vi "From Scratch.vi"() -> ()   [LabVIEW 2020]
uses:
  <vilib>/userdefined/High Color/IMAQdx.ctl
  <vilib>/vision/driver/IMAQdx.llb/IMAQdx Acquisition Mode.ctl
  <vilib>/vision/driver/IMAQdx.llb/IMAQdx Buffer Number Mode.ctl
  <vilib>/vision/driver/NI_Vision_Acquisition_Software.lvlib
  <resource>/objmgr/imaqdx.rc
panel:
  in  "Stop Stream":bool
  in  "Simulated Processing Delay (ms)":i32
  out "Buffer Number Out":u32
  out "Images Missed":u32
  out "Images Behind":i32
  out "Processed Frames per Second":dbl
  out "Acquired Frames per Second":dbl
  out "Image":T1(plugin-control)
  in  "Number of Images (err Iteration)":i32
  in  "OverwriteMode":u16(ring) items=["Get Oldest"=0, "Fail"=2, "Get Newest"=3]
  in  "IMAQdx Session":T2
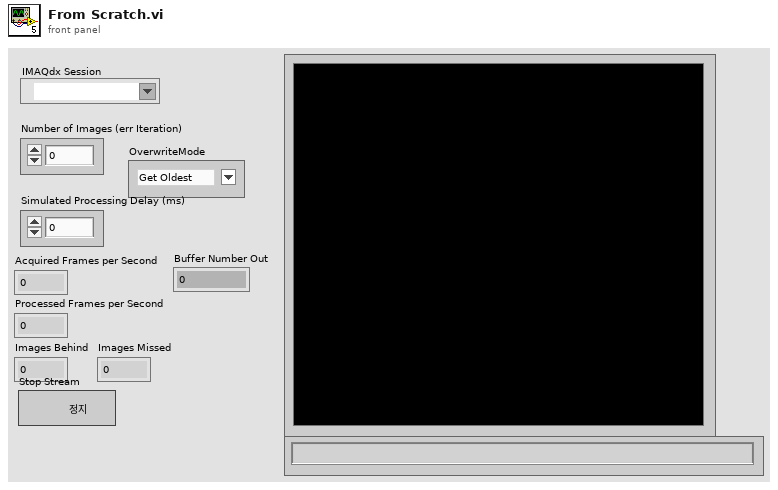
[diagram p1: front panel]
types:
  T1 = typedef "IMAQ Image.ctl" = refnum<image>
  T2 = typedef "IMAQdx.ctl" = refnum<k21>
  T3 = typedef "NI_Vision_Acquisition_Software.lvlib/IMAQdx Acquisition Mode.ctl" = enum32{"One Shot", "Continuous"}
  T4 = typedef "NI_Vision_Acquisition_Software.lvlib/IMAQdx Buffer Number Mode.ctl" = enum32{"Next", "Last", "Buffer Number", "Every", "Last New"}
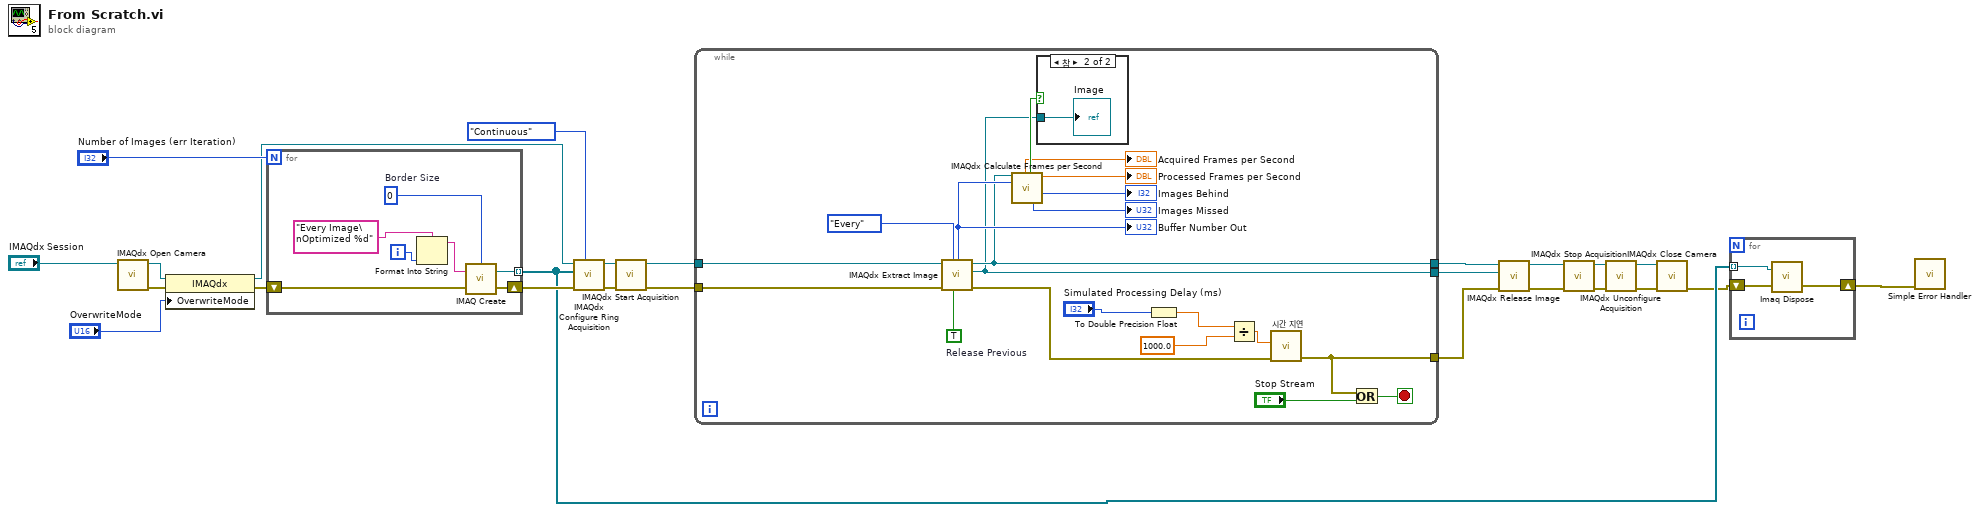
[diagram p0: block diagram]
diagram:
  n1 = call <vilib>:"IMAQdx Open Camera.vi"("Session In"="IMAQdx Session") -> ("error out"=w23:errorcluster, "Session Out"=w24:T2)  [unwired: 9 in]
  n2 = property class="IMAQdx"(reference=w24, error in=w23, "OverwriteMode"="OverwriteMode") -> (reference out=w18:T2, error out=w20:errorcluster)
  n3 = for {
    N: "Number of Images (err Iteration)" -> [_]
    tunnel: [w28] -> w3 mode=indexing
    shift-right: [w26] -> w17
    shift-left: w20 -> [w27]
    i -> [w31]
    w29 = 0  # Border Size
    n4 = Format Into String(format string="Every Image\nOptimized %d", w31) -> (resulting string=w30:string)  [unwired: 2 in, 1 out]
    n5 = call "IMAQ Create"("Border Size"=w29, "Image Name"=w30, "error in (no error)"=w27) -> ("New Image"=w28:T1, "error out"=w26:errorcluster)  [unwired: 2 in]
  }
  n6 = call <vilib>:"IMAQdx Configure Ring Acquisition.vi"("Mode"=IMAQdx_Acquisition_Mode."Continuous", "error in"=w17, "Images"=w3, "Session In"=w18) -> ("error out"=w15:errorcluster, "Session Out"=w16:T2)  [unwired: 5 in, 1 out]
  n7 = call <vilib>:"IMAQdx Start Acquisition.vi"("error in"=w15, "Session In"=w16) -> ("error out"=w14:errorcluster, "Session Out"=w13:T2)  [unwired: 8 in]
  n8 = while {
    tunnel: w14 -> [w38]
    tunnel: w13 -> [w52]
    tunnel: [w35] -> w10
    tunnel: [w34] -> w12
    tunnel: [w33] -> w11
    stop <- w41 stop-if-true
    w50 = TRUE  # Release Previous
    n9 = call <vilib>:"IMAQdx Extract Image.vi"("Release Previous (true)"=w50, "Buffer Number Mode (Next)"=IMAQdx_Buffer_Number_Mode."Every", "error in"=w38, "Session In"=w52) -> ("error out"=w47:errorcluster, "Buffer Number Out"=w49:u32, "Image Out"=w33:T1, "Session Out"=w34:T2)  [unwired: 4 in]
    "Buffer Number Out" <- w49
    n10 = call <vilib>:"IMAQdx Calculate Frames per Second.vi"("Session In"=w34, "Buffer Number"=w49) -> ("Update Display"=w48:bool, "Acquired Frames per Second"=→"Acquired Frames per Second":dbl, "Processed Frames per Second"=→"Processed Frames per Second":dbl, "Images Behind"=→"Images Behind":i32, "Images Missed"=→"Images Missed":u32)  [unwired: 7 in, 2 out]
    n11 = case shown="참" w48 {
      tunnel: w33 -> [_ w53]
      frame False {
      }
      frame True {
        "Image" <- w53
      }
    }
    n12 = To Double Precision Float(number="Simulated Processing Delay (ms)") -> (double precision float=w37:dbl)
    n13 = Divide(x=w37, y=1000.0) -> (x/y=w42:dbl)
    n14 = call "시간 지연"("error in (no error)"=w47, "Delay Time (s)"=w42) -> ("error out"=w35:errorcluster)  [unwired: 9 in]
    n15 = Or(x=w35, y="Stop Stream") -> (x .or. y?=w41:bool)
  }
  n16 = call <vilib>:"IMAQdx Release Image.vi"("error in"=w10, "Image"=w11, "Session In"=w12) -> ("error out"=w8:errorcluster, "Session Out"=w9:T2)  [unwired: 7 in]
  n17 = call <vilib>:"IMAQdx Stop Acquisition.vi"("error in"=w8, "Session In"=w9) -> ("error out"=w7:errorcluster, "Session Out"=w6:T2)  [unwired: 8 in]
  n18 = call <vilib>:"IMAQdx Unconfigure Acquisition.vi"("error in"=w7, "Session In"=w6) -> ("error out"=w4:errorcluster, "Session Out"=w5:T2)  [unwired: 8 in]
  n19 = call <vilib>:"IMAQdx Close Camera.vi"("error in"=w4, "Session In"=w5) -> ("error out"=w1:errorcluster)  [unwired: 9 in]
  n20 = for {
    tunnel: w3 -> [w56] mode=indexing
    shift-right: [w55] -> w2
    shift-left: w1 -> [w54]
    n21 = call "Imaq Dispose"("Image"=w56, "error in (no error)"=w54) -> ("error out"=w55:errorcluster)  [unwired: 4 in]
  }
  n22 = call <vilib>:"Simple Error Handler.vi"("error in (no error)"=w2) -> ()  [unwired: 4 in, 5 out]
